vi "Reorder Keys.vi"(10 "Test Registrations in":T1[](array[typedef]), 11 "Keys in":string[](array[string])) -> (2 "Test Registrations out":T1[](array[typedef]), 3 "Keys out":string[](array[string]))   [LabVIEW 2013, in "Caraya.lvlib" / "Basic Test Manager.lvclass"]
uses:
  Basic Test Manager.lvclass
  Test Result/Test Node.ctl
  Test Result/Test Registration Data.ctl
  Test Result/Test Result.lvclass
panel:
  out "Ordered Keys":string[](array[string])
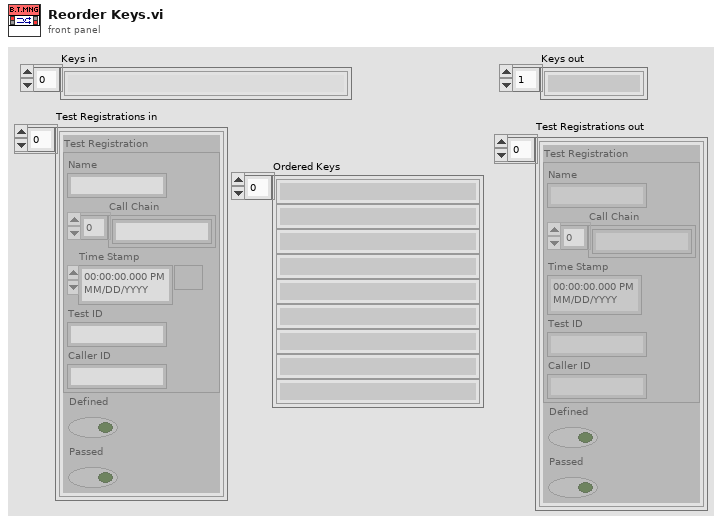
[diagram p1: front panel]
types:
  T1 = typedef "Caraya.lvlib/Test Result.lvclass/Test Node.ctl" = cluster{"Test Registration":T2, "Defined":bool, "Passed":bool}
  T2 = typedef "Caraya.lvlib/Test Result.lvclass/Test Registration Data.ctl" = cluster{"Name":string, "Call Chain":string[], "Time Stamp":timestamp, "Test ID":string, "Caller ID":string}
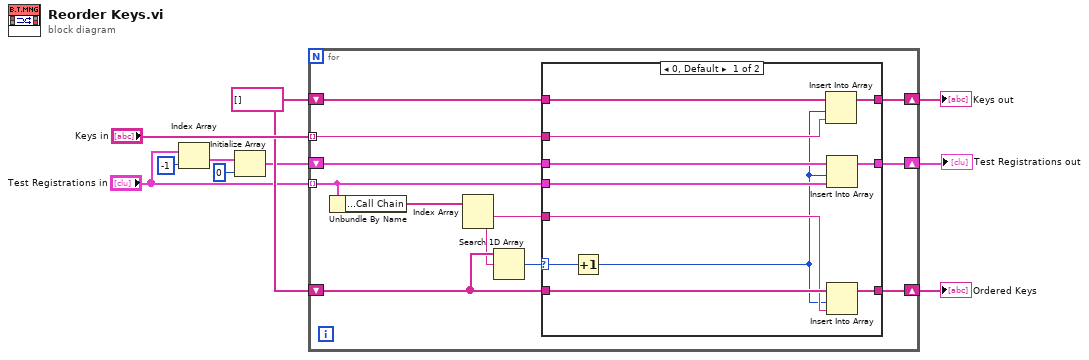
[diagram p0: block diagram]
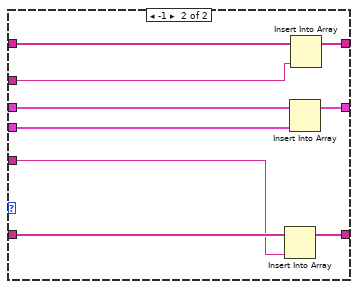
[diagram p2: hidden frame]
diagram:
  w7 = string[] [] ("Keys out")
  n1 = Index Array(array="Test Registrations in", index=-1) -> (element=w5:T1)
  n2 = Initialize Array(w5, 0 ("dimension size")) -> (w3:T1[])
  n3 = for {
    tunnel: "Keys in" -> [w16] mode=indexing
    tunnel: "Test Registrations in" -> [w11] mode=indexing
    shift-right: [w19] -> w9
    shift-left: w7 -> [w20]
    shift-right: [w17] -> w1
    shift-left: w3 -> [w18]
    shift-right: [w21] -> w8
    shift-left: w7 -> [w22]
    n4 = Unbundle By Name(w11) -> ("Test Registration.Call Chain"=w12:string[])
    n5 = Index Array(array=w12) -> (element #1=w14:string, element #2=w13:string)  [unwired: 2 in]
    n6 = Search 1D Array(1D array=w22, element=w13) -> (index of element=w15:i32)  [unwired: 1 in]
    n7 = case shown="0, Default" w15 {
      selector: w15 -> [w24 _]
      tunnel: w22 -> [w33 w42]
      tunnel: w14 -> [w31 w41]
      tunnel: [w32 w40] -> w21
      tunnel: w20 -> [w30 w39]
      tunnel: [w29 w38] -> w19
      tunnel: w18 -> [w25 w37]
      tunnel: [w28 w36] -> w17
      tunnel: w16 -> [w27 w35]
      tunnel: w11 -> [w26 w34]
      frame 0, Default {
        n8 = Increment(x=w24) -> (x+1=w23:i32)
        n9 = Insert Into Array(array=w30, index=w23, new element=w27) -> (w29:string[])
        n10 = Insert Into Array(array=w25, index=w23, new element=w26) -> (w28:T1[])
        n11 = Insert Into Array(array=w33, index=w23, new element=w31) -> (w32:string[])
      }
      frame -1 {
        n12 = Insert Into Array(array=w42, new element=w41) -> (w40:string[])  [unwired: 1 in]
        n13 = Insert Into Array(array=w37, new element=w34) -> (w36:T1[])  [unwired: 1 in]
        n14 = Insert Into Array(array=w39, new element=w35) -> (w38:string[])  [unwired: 1 in]
      }
    }
  }
  "Keys out" <- w9
  "Test Registrations out" <- w1
  "Ordered Keys" <- w8
